vi "FileErrorHandler.vi"(0 "EpiWrapper in":refnum<class "EpiWrapper.lvclass">, 1 "FilePathErrors":errorcluster[](array[cluster]), 2 "error in (no error)":errorcluster) -> (3 "EpiWrapper out":refnum<class "EpiWrapper.lvclass">, 4 "ErrorActions":T1, 5 "Error Message":string, 6 "error out":errorcluster)   [LabVIEW 2012, in "EpiWrapper.lvclass"]
uses:
  EpiWrapper.lvclass
  Controls/ErrorActions.ctl
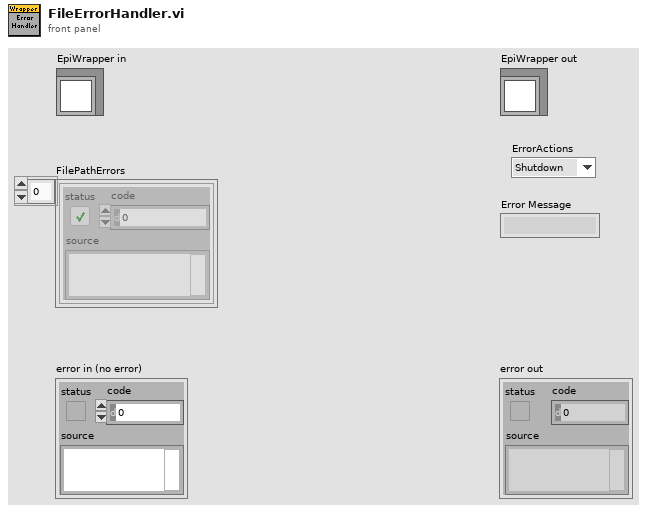
[diagram p1: front panel]
types:
  T1 = typedef "ErrorActions.ctl" = enum16{"Shutdown", "Warning", "Reset", "NoAction"}
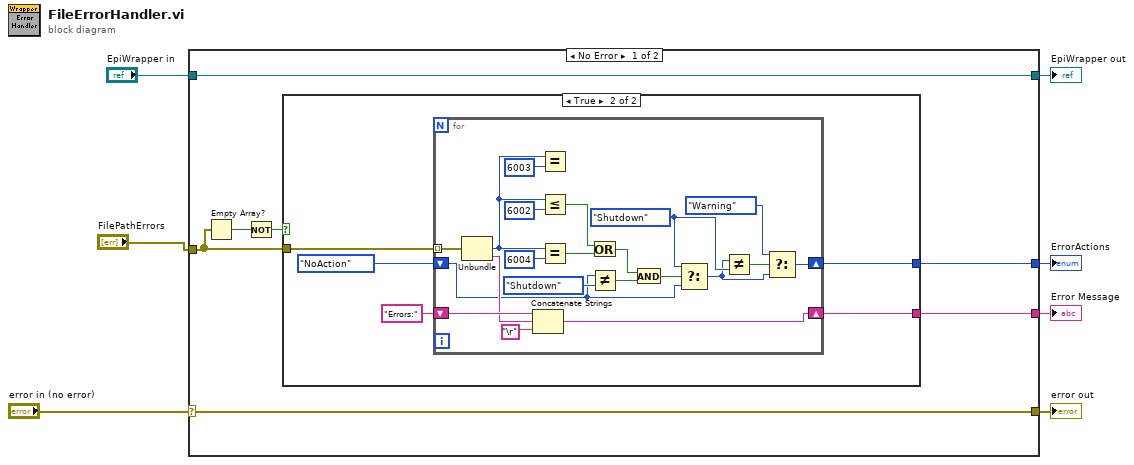
[diagram p0: block diagram]
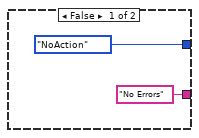
[diagram p2: hidden frame]
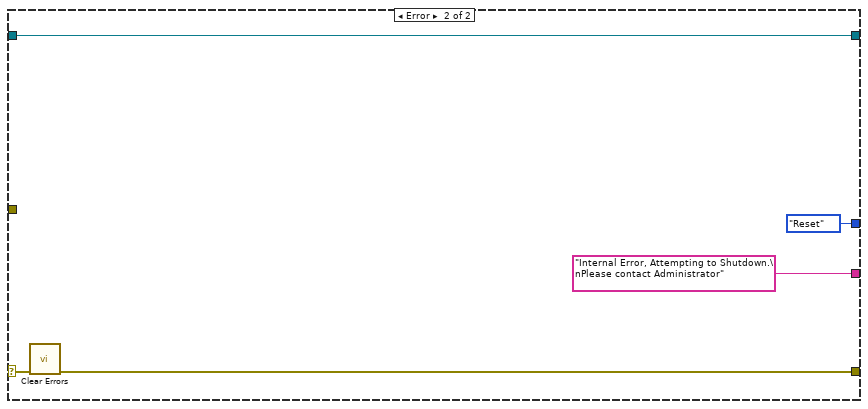
[diagram p3: hidden frame]
diagram:
  n1 = case shown="No Error" "error in (no error)" {
    selector: "error in (no error)" -> [w13 w46]
    tunnel: [w13 w45] -> w6
    tunnel: [w14 w47] -> w4
    tunnel: "EpiWrapper in" -> [w14 w47]
    tunnel: "FilePathErrors" -> [w9 _]
    tunnel: [w10 ErrorActions."Reset" ("ErrorActions")] -> w2
    tunnel: [w8 "Internal Error, Attempting to Shutdown.\nPlease contact Administrator"] -> w1
    frame No Error {
      n2 = Empty Array?(array=w9) -> (empty?=w12:bool)
      n3 = Not(x=w12) -> (.not. x?=w11:bool)
      n4 = case shown="True" w11 {
        tunnel: [ErrorActions."NoAction" ("ErrorActions") w17] -> w10
        tunnel: w9 -> [_ w21]
        tunnel: ["No Errors" w19] -> w8
        frame False {
        }
        frame True {
          n5 = for {
            tunnel: w21 -> [w42] mode=indexing
            shift-right: [w32] -> w19
            shift-left: "Errors:" -> [w35]
            shift-right: [w22] -> w17
            shift-left: ErrorActions."NoAction" ("ErrorActions") -> [w27]
            w26 = ErrorActions."Shutdown" ("ErrorActions")
            n6 = Unbundle(w42) -> ("code"=w37:i32, "source"=w34:string)  [unwired: 1 out]
            n7 = Concatenate Strings(w35, w34, "\r") -> (w32:string)
            n8 = Equal?(x=w37, y=6003) -> ()  [unwired: 1 out]
            n9 = Less Or Equal?(x=w37, y=6002) -> (x <= y?=w40:bool)
            n10 = Equal?(x=w37, y=6004) -> (x = y?=w38:bool)
            n11 = Or(x=w40, y=w38) -> (x .or. y?=w29:bool)
            n12 = Not Equal?(x=w27, y=ErrorActions."Shutdown" ("ErrorActions")) -> (x != y?=w30:bool)
            n13 = And(x=w29, y=w30) -> (x .and. y?=w28:bool)
            n14 = Select(t=w26, s=w28, f=w27) -> (s? t:f=w24:T1)
            n15 = Not Equal?(x=w24, y=w26) -> (x != y?=w25:bool)
            n16 = Select(t=ErrorActions."Warning", s=w25, f=w24) -> (s? t:f=w22:T1)
          }
        }
      }
    }
    frame Error {
      n17 = call <vilib>:"Clear Errors.vi"("error in (no error)"=w46) -> ("error out"=w45:errorcluster)  [unwired: 6 in]
    }
  }
  "error out" <- w6
  "EpiWrapper out" <- w4
  "ErrorActions" <- w2
  "Error Message" <- w1
